vi "fpga_transmission_control_3V10.vi"() -> ()   [LabVIEW 2017]
uses:
  Control 1.ctl
  <vilib>/Platform/TimedLoop/XDataNode/timing_clust.ctl
  <vilib>/Platform/TimedLoop/XDataNode/nitl_modes.ctl
  <vilib>/Platform/TimedLoop/XDataNode/wakeup.ctl
  <vilib>/Instr/_visa.llb/VISA Configure Serial Port (Serial Instr).vi
  <vilib>/platform/TimedLoop/XDataNode/XDataNode.xnode
  <vilib>/Platform/TimedLoop/XDataNode/XDNodeRunTimeDep.lvlib
panel:
  out "Timer":dbl
  out "Output":bool
  out "outcome":u32
  out "currentType":string
  out "Time":dbl(slide) scale=0.0..100.0
  out "Progress":dbl(slide) scale=0.0..100.0
  in  "error in (no error)":errorcluster
  out "PWM":bool
  out "pattern":u32
  in  "Timeslot":bool
  out "type":string
  out "Kombi Chart":cluster{u16, i16}(graph)
  out "contingency":string
  in  "Array":T2(array[cluster]) {"duration" step=1}
  out "Timeslot":i32
  out "Sign":bool
  out "deleted portion":u8[](array[numeric])
  out "data":bool
  out "x-y":u16
  out "Error String":string
  out "error out":errorcluster
  out "Timing":u32
  out "Int_pixel":i16
  out "Pixel":u16(graph)
  out "AD_Value":i16
  in  "millisecond timer value 2":u32
  out "AD_Chart":i16(graph)
  in  "Path":path
  out "Read":bool
  in  "Stop Program":bool
  in  "Start":bool
  in  "VISA resource name":refnum<visa-resource-name>
  # "UR Elektronik Biologie\nTerminal V 3.8"
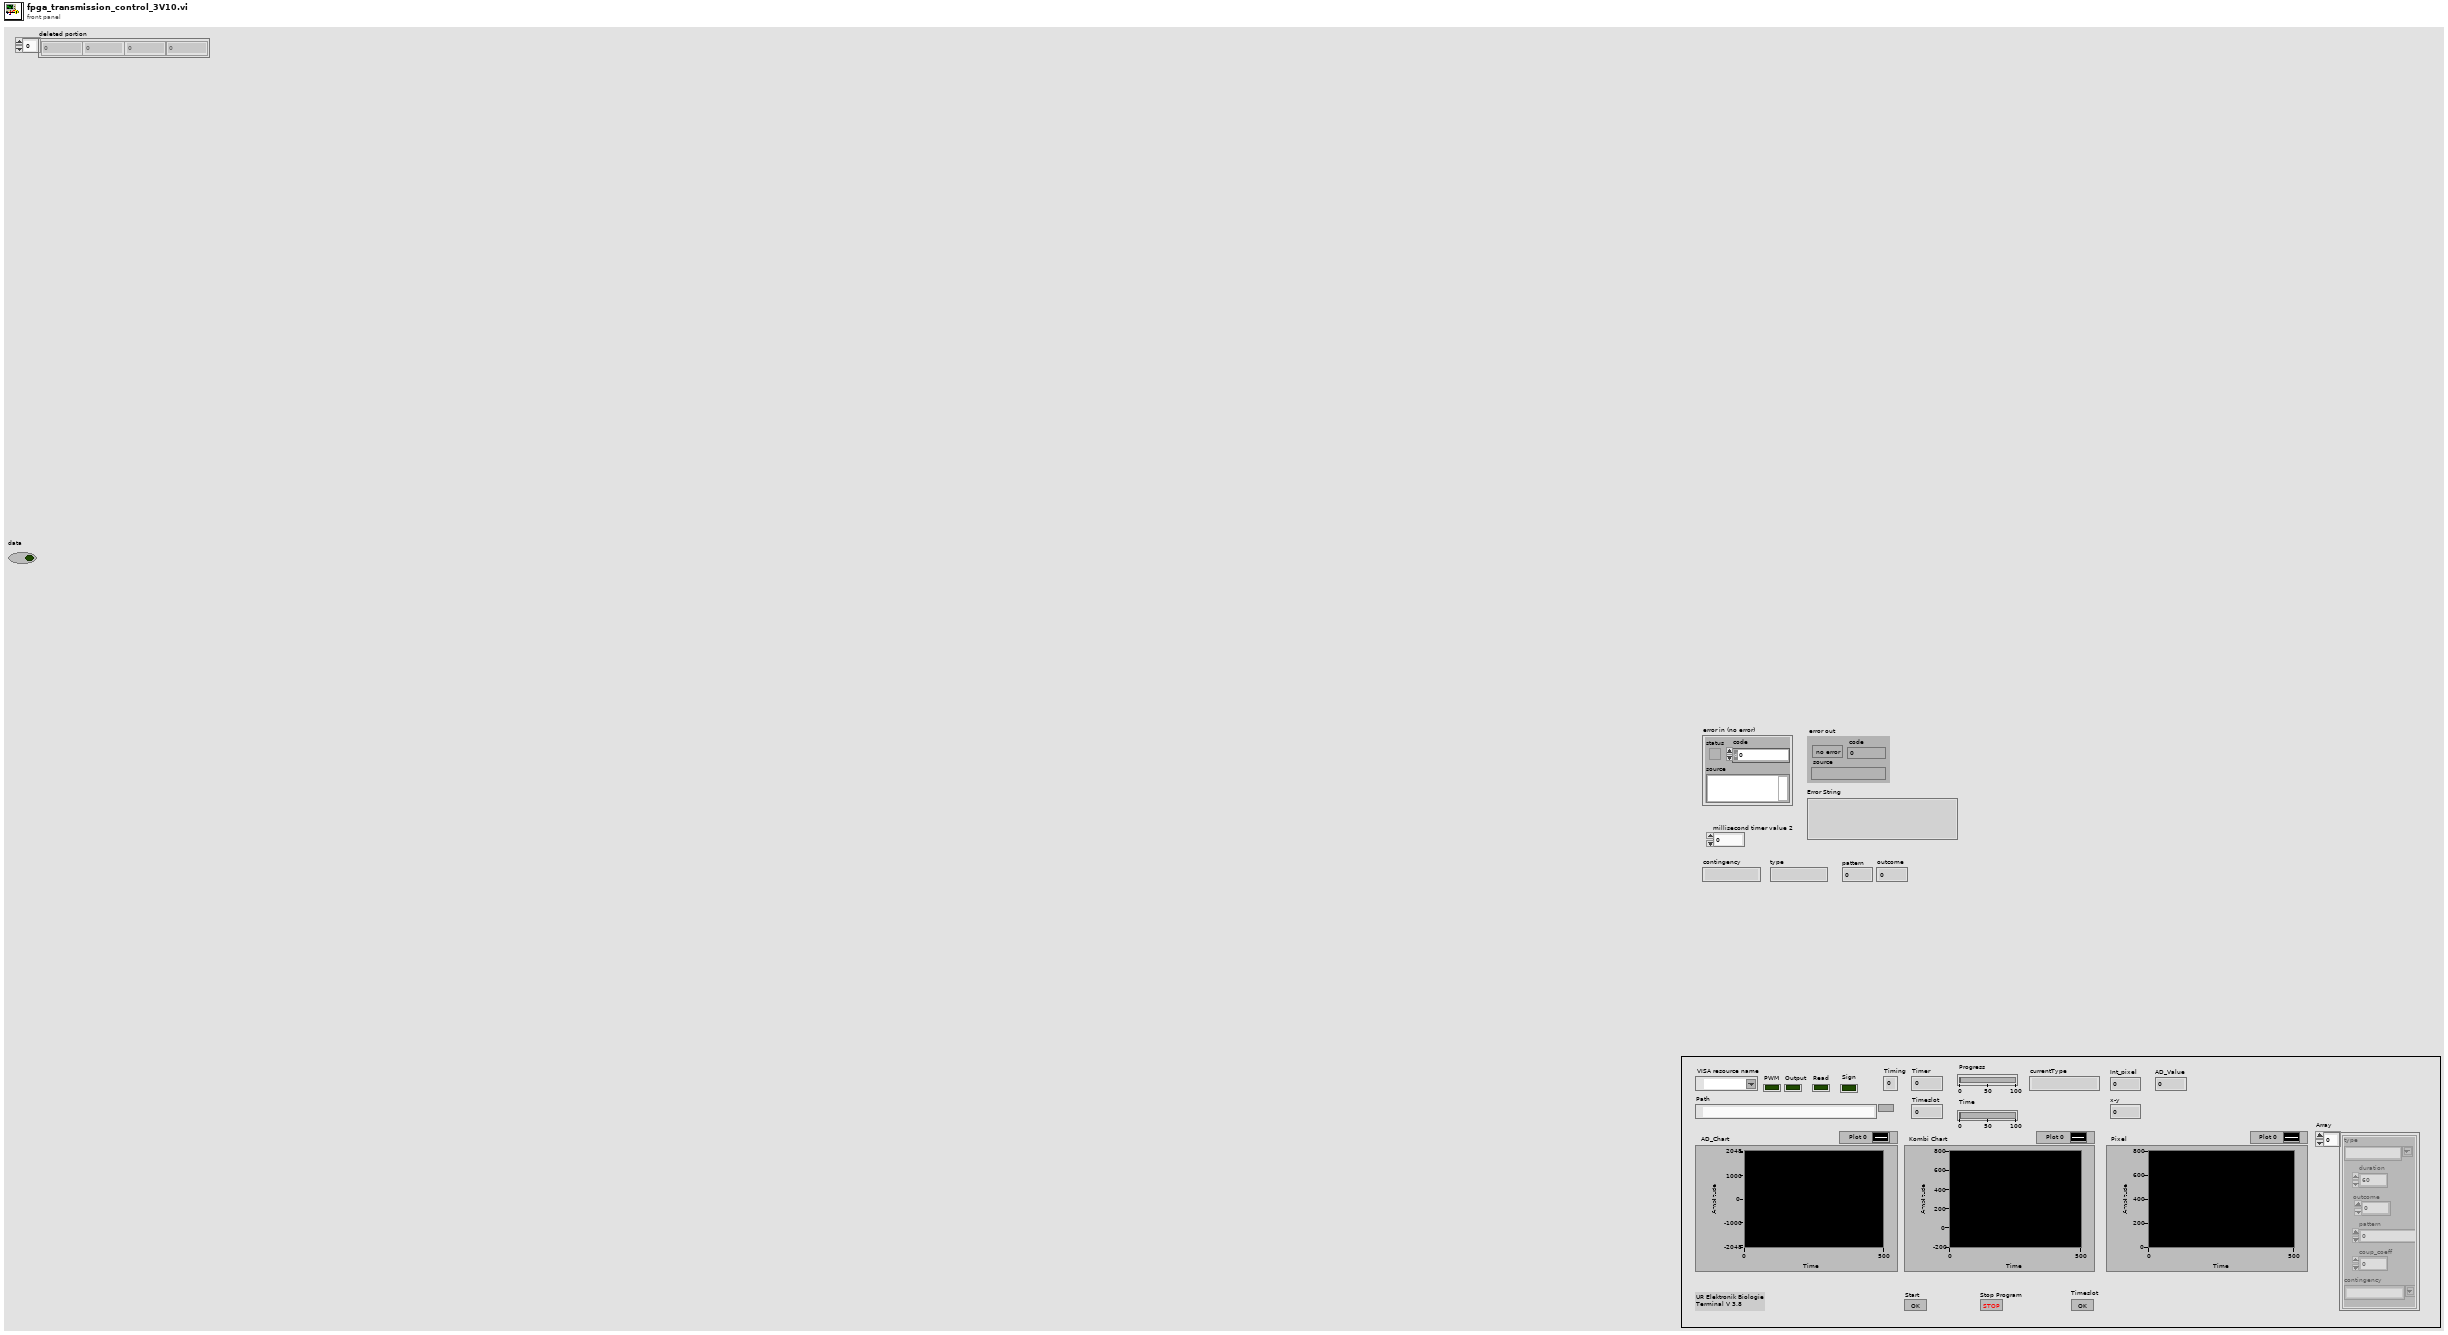
[diagram p1: front panel]
types:
  T1 = typedef "Control 1.ctl" = u32
  T2 = cluster{"type":string, "duration":T1, "outcome":u32, "pattern":u32, "coup_coeff":u32, "contingency":string}[]
  T3 = typedef "XDNodeRunTimeDep.lvlib/timing_clust.ctl" = cluster{"Expected End [f-1]":u64, "Actual End [f-1]":u64, "Finished Late? [f-1]":bool, "Expected End [i-1]":u64, "Actual End [i-1]":u64, "Finished Late? [i-1]":bool, "Expected Start [i]":u64, "Actual Start [i]":u64, "Expected Start [f]":u64, "Actual Start [f]":u64, "Source Name":string, "Structure Name":string, "Period":i64, "Deadline":i64, "Offset":i64, "Start":i64, "Priority":i32, "Timeout":i32, "Mode":T4, "Wakeup Reason":T5, "Error":errorcluster, "Source Type":string, "Secondary Source Type":string, "Global End Time":u64, "Global Start Time":u64, "Frame Duration":u64, "Iteration Duration":u64, "Assigned CPU":i32, "I/O Scan Engine Mode":u32}
  T4 = typedef "XDNodeRunTimeDep.lvlib/nitl_modes.ctl" = enum32{"No Change", "Process missed periods, maintain original phase", "Discard missed periods, maintain original phase", "Process missed periods, ignore original phase", "Discard missed periods, ignore original phase"}
  T5 = typedef "XDNodeRunTimeDep.lvlib/wakeup.ctl" = enum32{"Normal", "Aborted", "Asynchronous wakeup", "Timing source error", "Timed loop error", "Timeout"}
  T6 = cluster{"String":string, i32, i32, u32, u32, "String":string}[]
  T7 = enum16{"Idel", "State1", "State2", "State3", "State4"}
  T8 = enum16{"open", "replace", "create", "open or create", "replace or create", "replace or create with confirmation"}
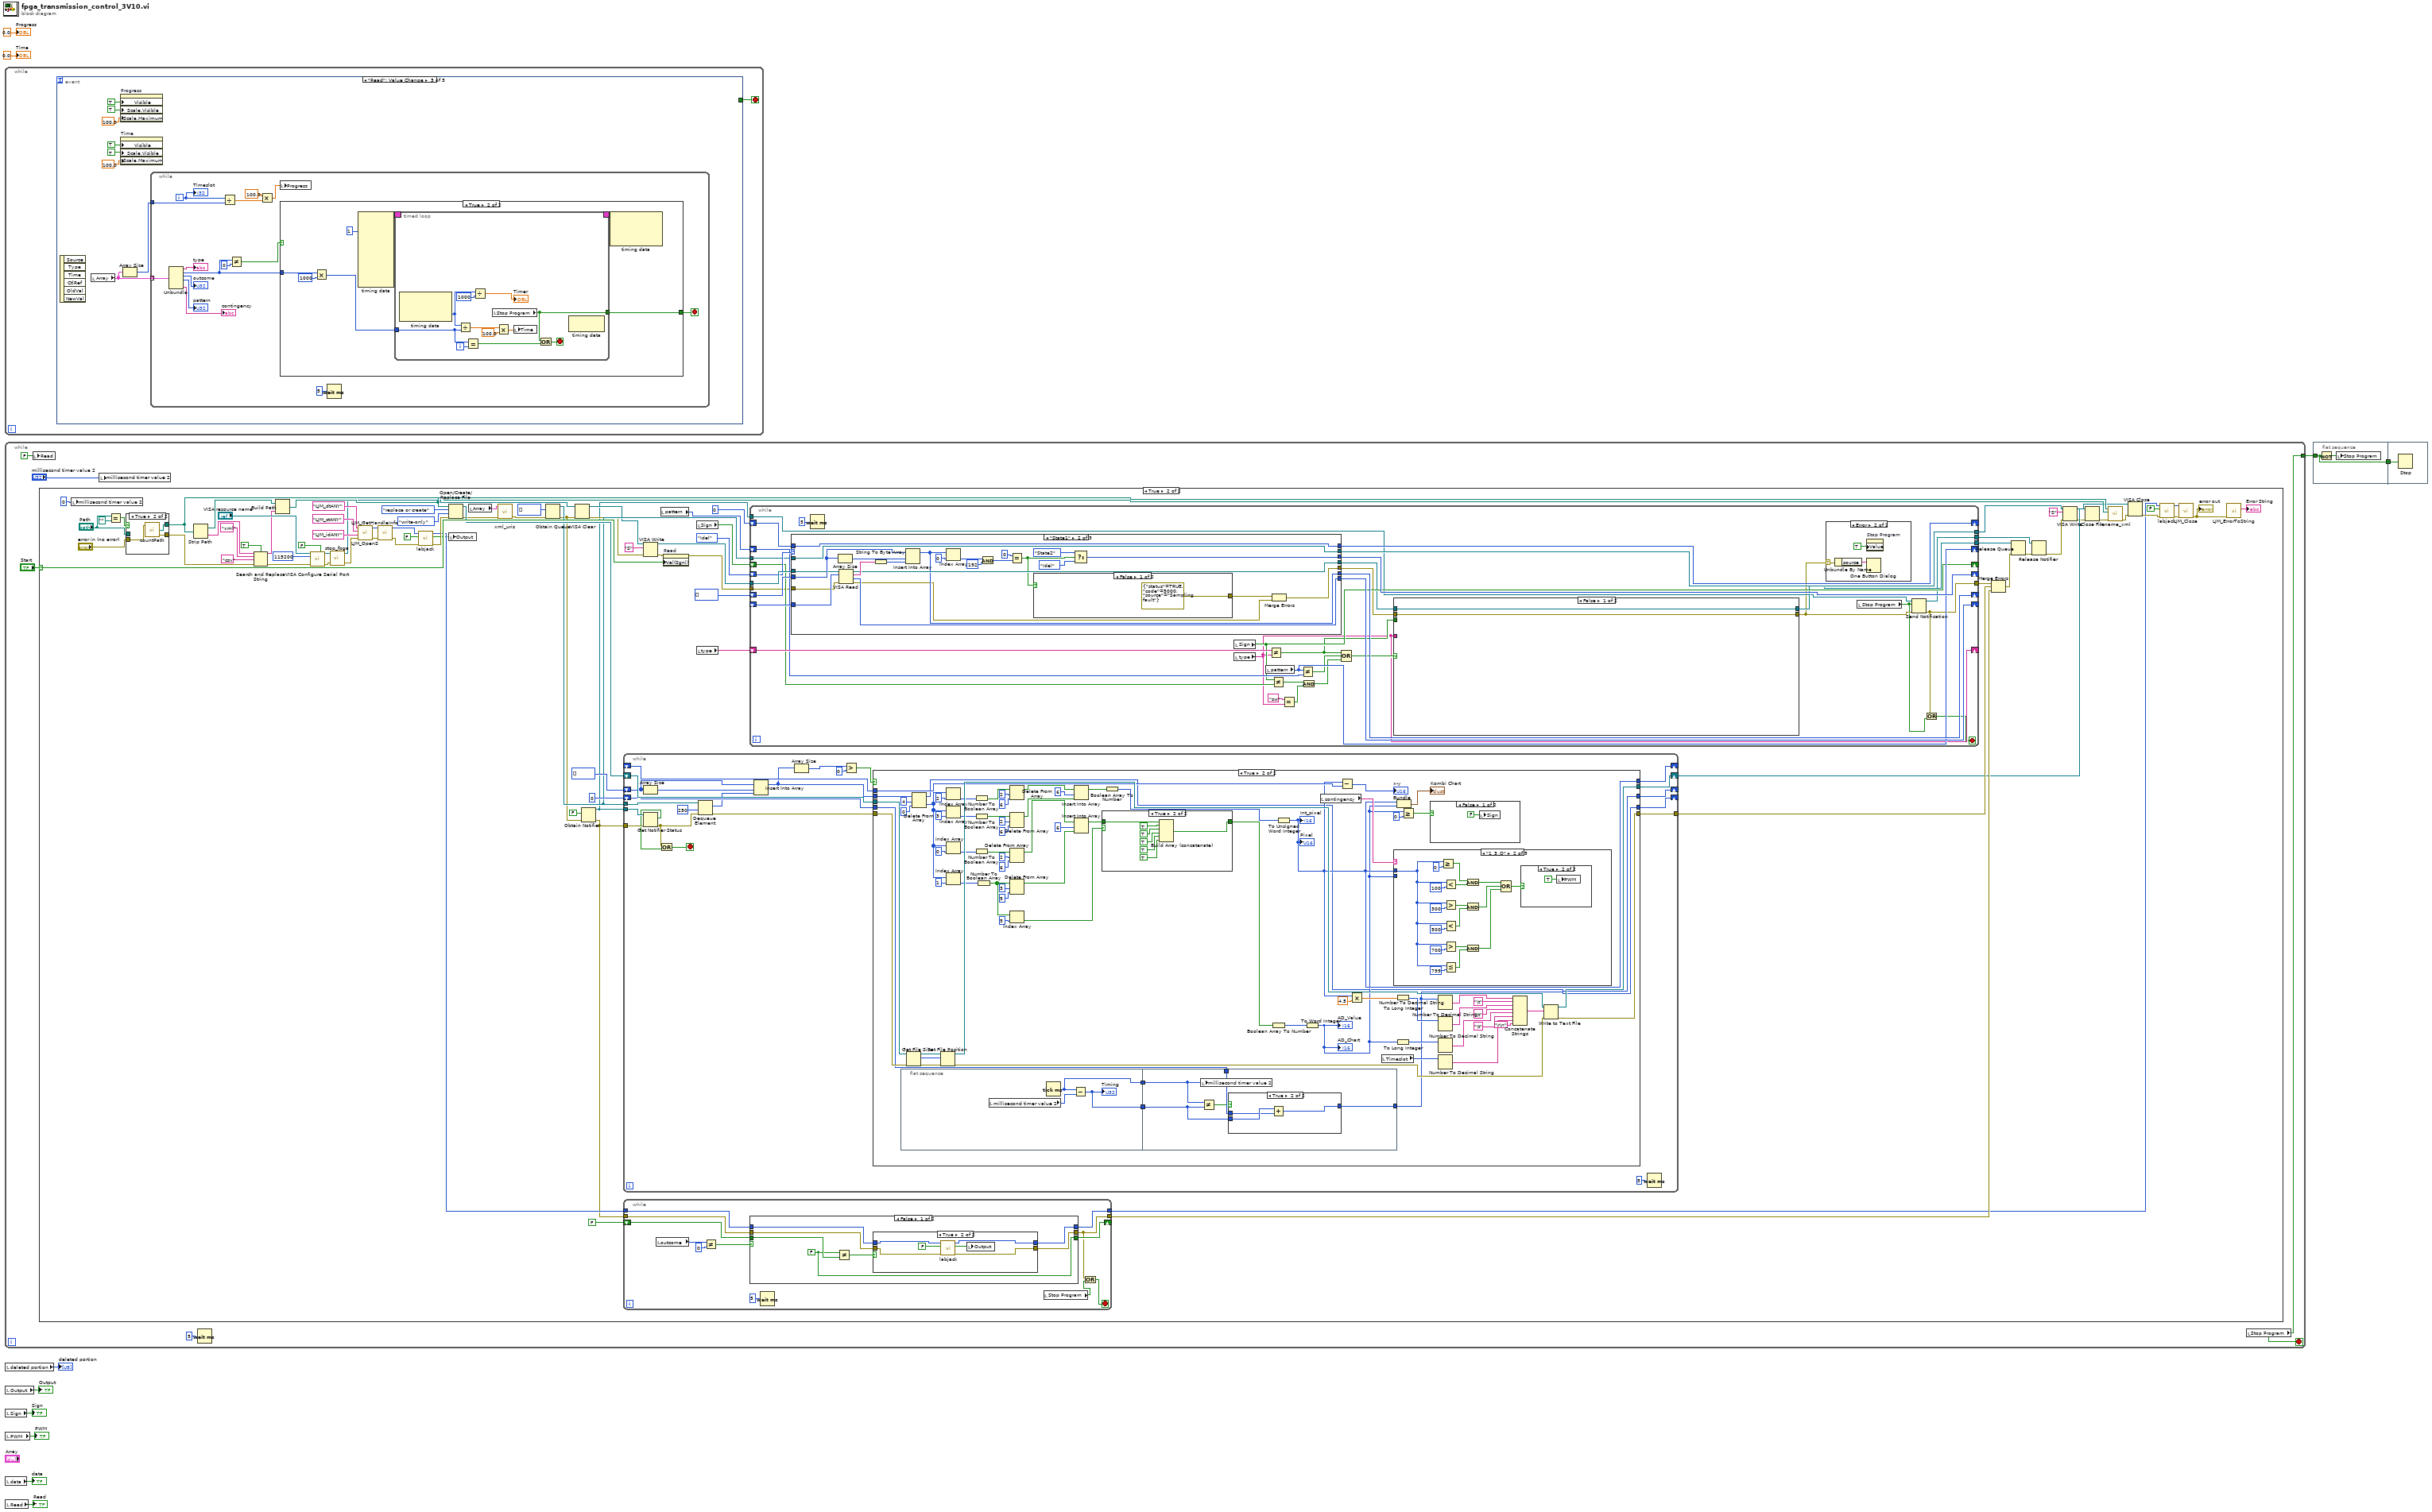
[diagram p0: block diagram]
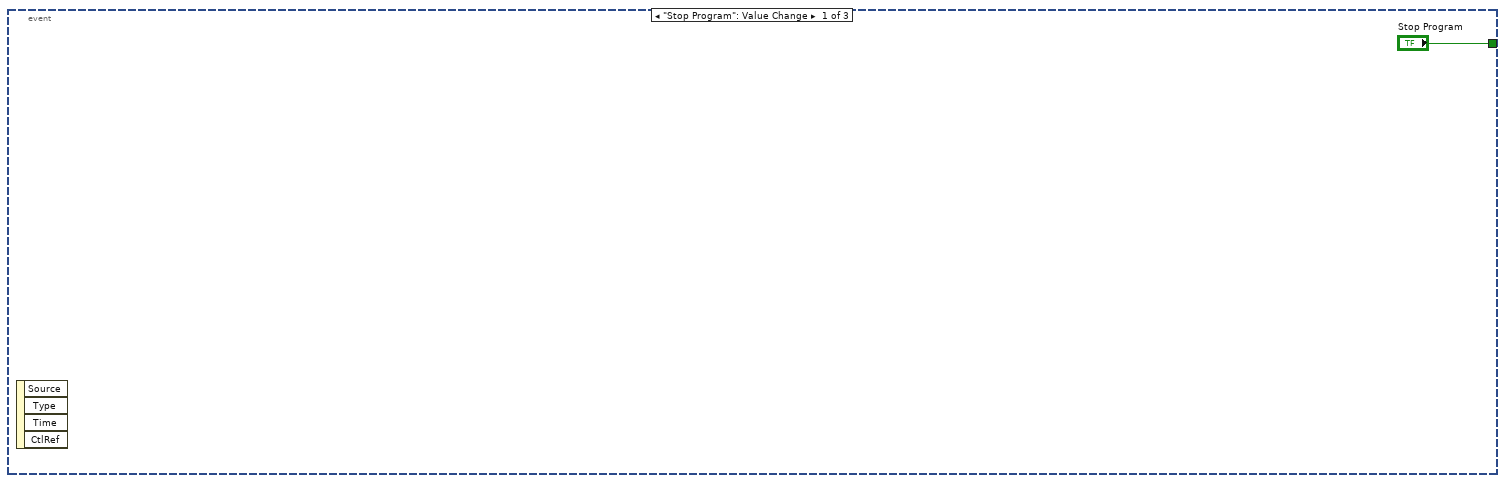
[diagram p2: hidden frame]
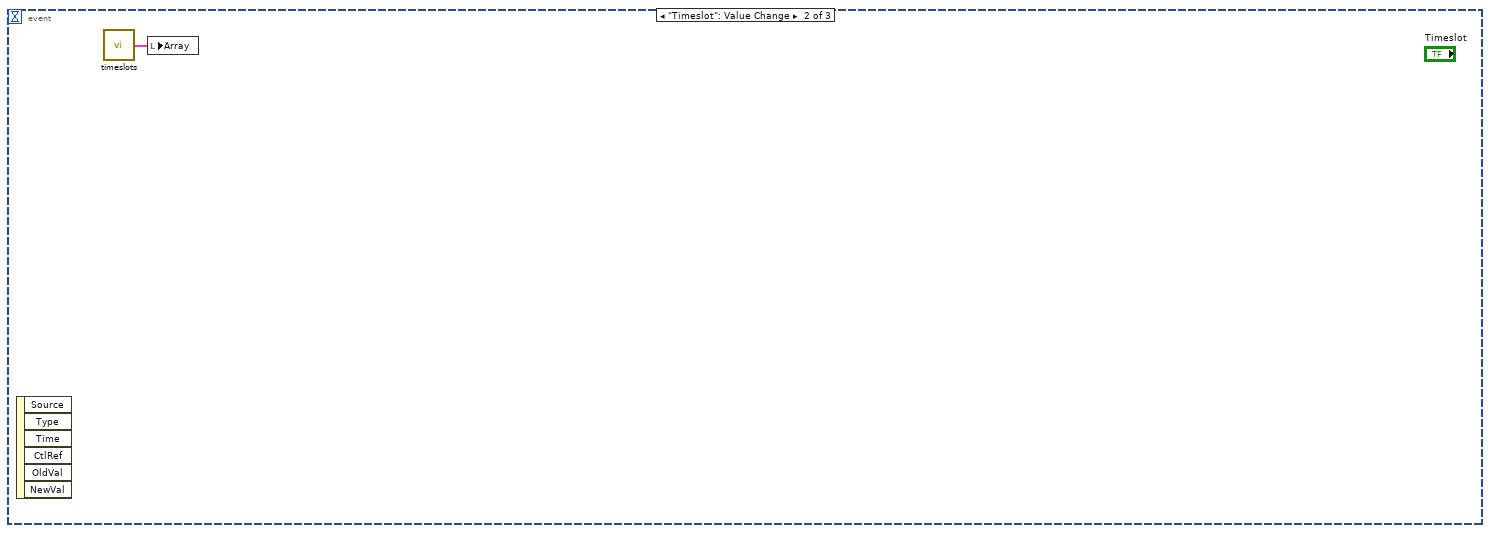
[diagram p3: hidden frame]
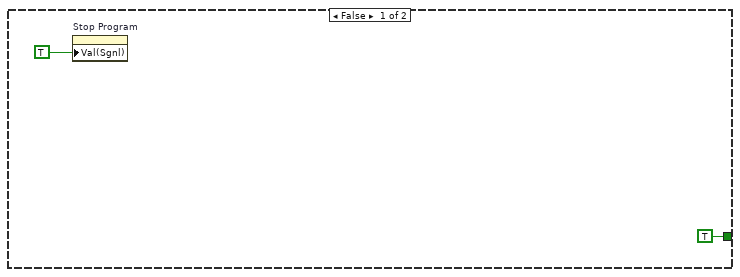
[diagram p4: hidden frame]
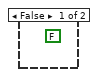
[diagram p5: hidden frame]
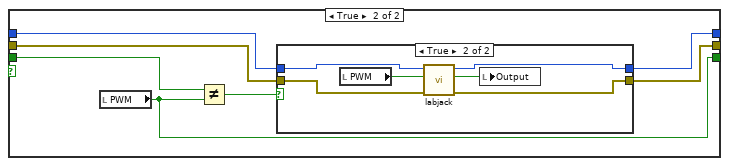
[diagram p8: hidden frame]
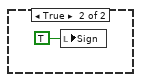
[diagram p11: hidden frame]
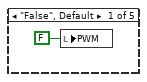
[diagram p12: hidden frame]
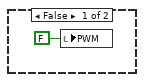
[diagram p13: hidden frame]
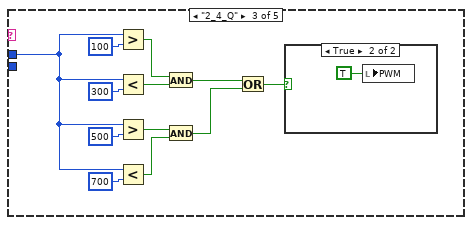
[diagram p14: hidden frame]
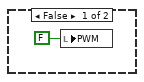
[diagram p15: hidden frame]
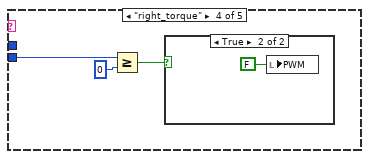
[diagram p16: hidden frame]
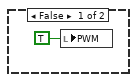
[diagram p17: hidden frame]
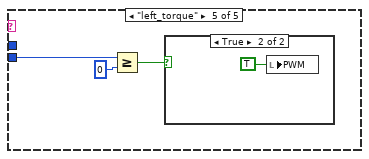
[diagram p18: hidden frame]
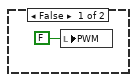
[diagram p19: hidden frame]
diagram:
  n1 = while {
    stop <- w11 stop-if-true
    n2 = event shown="[2] \"Read\": Value Change" {
      selector: _ -> [_ _ _]
      dyn-events: _ -> [_ _ _]
      timeout: _ -> [_ _ _]
      tunnel: ["Stop Program" _ _] -> w11
      event "Stop Program": Value Change {
        n3 = event-data() -> ()  [unwired: 1 in, 4 out]
      }
      event "Timeslot": Value Change {
        n4 = event-data() -> ()  [unwired: 1 in, 6 out]
        n5 = call "timeslots.vi"() -> ("array of clusters"=w13:T6)  [unwired: 1 in, 1 out]
        n6 = local write "Array"(w13) -> ()
      }
      event "Read": Value Change {
        n7 = event-data() -> ()  [unwired: 1 in, 6 out]
        n8 = local read "Array"() -> (w21:T2)
        n9 = property on="Progress" class="Slide (strict)"("Visible"=TRUE, "Scale.Visible"=TRUE ("Visible"), "Scale.Maximum"=100.0 ("Scale.Range:Maximum")) -> ()  [unwired: 2 in, 2 out]
        n10 = property on="Time" class="Slide (strict)"("Visible"=TRUE, "Scale.Visible"=TRUE ("Visible"), "Scale.Maximum"=100.0 ("Scale.Range:Maximum")) -> ()  [unwired: 2 in, 2 out]
        n11 = Array Size(array=w21) -> (size(s)=w20:i32)
        n12 = while {
          tunnel: w21 -> [w36] mode=indexing
          tunnel: w20 -> [w29]
          i -> [w28]
          stop <- w22 stop-if-true
          n13 = Unbundle(w36) -> ("type"=→"type":string, "duration"=w23:T1, "outcome"=→"outcome":u32, "pattern"=→"pattern":u32, "contingency"=→"contingency":string)  [unwired: 1 out]
          n14 = Divide(x=w28, y=w29) -> (x/y=w27:dbl)
          n15 = Not Equal?(x=w23, y=u32 0) -> (x != y?=w34:bool)
          n16 = Multiply(x=100.0 ("y"), y=w27) -> (x*y=w25:dbl)
          n17 = local write "Progress"(w25) -> ()
          n18 = case shown="True" w34 {
            tunnel: w23 -> [_ w42]
            tunnel: [TRUE w39] -> w22
            frame False {
              n19 = property on="Stop Program" class="Bool (strict)"("Val(Sgnl)"=TRUE) -> ()  [unwired: 2 in, 2 out]
            }
            frame True {
              n20 = Multiply(x=w42, y=T1 1000) -> (x*y=w40:T1)
              n21 = node-c288(i64 1 ("Period")) -> (w45:T3)  [unwired: 8 in]
              n22 = timed-loop {
                timing: w45 -> [_]
                timing-out: [_] -> w44
                tunnel: w40 -> [w52]
                tunnel: [w53] -> w39
                i -> [w56]
                stop <- w55 stop-if-true
                n23 = node-c288() -> (w48:i64)  [unwired: 1 in, 2 out]
                n24 = Divide(x=w48, y=w52) -> (x/y=w50:dbl)
                n25 = Equal?(x=w52, y=w56) -> (x = y?=w54:bool)
                n26 = Divide(x=w48, y=i64 1000) -> (x/y=→"Timer":dbl)
                n27 = local read "Stop Program"() -> (w53:bool)
                n28 = Multiply(x=w50, y=100.0) -> (x*y=w51:dbl)
                n29 = local write "Time"(w51) -> ()
                n30 = Or(x=w53, y=w54) -> (x .or. y?=w55:bool)
                n31 = node-c288() -> ()  [unwired: 1 in, 1 out]
              }
              n32 = node-c288(w44) -> ()  [unwired: 3 out]
            }
          }
          n33 = Wait (ms)(milliseconds to wait=u32 5) -> ()  [unwired: 1 out]
          "Timeslot" <- w28
        }
      }
    }
  }
  n34 = while {
    tunnel: [w67] -> w10
    stop <- w67 stop-if-true
    n35 = local write "Read"(FALSE) -> ()
    n36 = case shown="True" "Start" {
      selector: "Start" -> [_ w145]
      frame False {
        (unwired) FALSE
      }
      frame True {
        n37 = local write "millisecond timer value 2"(u32 0 ("millisecond timer value 2")) -> ()
        n38 = Equal?(x="Path", y=path "") -> (x = y?=w132:bool)
        n39 = case shown="True" w132 {
          tunnel: [w153 w156] -> w98
          tunnel: "Path" -> [w153 _]
          tunnel: [w152 w155] -> w107
          tunnel: "error in (no error)" -> [w152 w154]
          frame False {
          }
          frame True {
            n40 = call "countPath.vi"("error in (no error)"=w154) -> ("error out"=w155:errorcluster, "appended path"=w156:path)
          }
        }
        n41 = Strip Path(path=w98) -> (stripped path=w111:path, name=w110:string)
        n42 = Search and Replace String(case sensitive?=TRUE ("ignore case? (F)"), input string=w110, search string="xml", replace string="csv" ("replace string (\"\")"), error in=w107) -> (result string=w104:string, error out=w106:errorcluster)  [unwired: 3 in, 2 out]
        n43 = Build Path(base path=w111, name or relative path=w104) -> (appended path=w99:path)
        n44 = call-poly "VISA Configure Serial Port"("VISA resource name"="VISA resource name", "Enable Termination\nChar (T)"=FALSE ("Enable Termination\nChar (T)"), "baud rate (9600)"=u32 115200, "error in (no error)"=w106) -> ("VISA resource name out"=w91:refnum<visa-resource-name>, "error out"=w90:errorcluster)  [unwired: 10 in]
        n45 = call "stop_fpga.vi"("error in (no error)"=w90, "reference"=w91) -> ("error out"=w89:errorcluster, "VISA resource name out"=w82:refnum<visa-resource-name>)  [unwired: 2 in]
        n46 = call "LJM_OpenS.vi"("error in"=w89, "Identifier"="LJM_idANY", "ConnectionType"="LJM_ctANY", "DeviceType"="LJM_dtANY") -> ("error out"=w135:errorcluster, "Handle"=w134:i32)  [unwired: 6 in]
        n47 = call "LJM_GetHandleInfo.vi"("error in"=w135, "Handle In"=w134) -> ("error out"=w137:errorcluster, "Handle Out"=w136:i32)  [unwired: 2 in, 6 out]
        n48 = call "labjack.vi"("error out"=w137, "Boolean"=FALSE, "Handle Out"=w136) -> ("error out 2"=w140:errorcluster, "Boolean 2"=w97:bool, "Handle Out 2"=w139:i32)  [unwired: 6 in]
        n49 = Open/Create/Replace File(file path (use dialog)=w99, error in=w140, operation (0:open)=T8."replace or create", access (0:read/write)=enum16{"read/write", "read-only", "write-only"}."write-only") -> (refnum out=w114:refnum<file>, error out=w112:errorcluster)  [unwired: 2 in, 1 out]
        n50 = local write "Output"(w97) -> ()
        n51 = local read "Array"() -> (w113:T2)
        n52 = call "xml_uris.vi"("error in"=w112, "Array"=w113) -> ("error out"=w83:errorcluster)  [unwired: 2 in, 2 out]
        n53 = Obtain Queue(element data type=u8[] [], error in (no error)=w83) -> (queue out=w85:refnum<queue>, error out=w70:errorcluster)  [unwired: 3 in, 1 out]
        n54 = VISA Clear(VISA resource name=w82, error in (no error)=w70) -> (VISA resource name out=w81:refnum<visa-resource-name>, error out=w79:errorcluster)
        n55 = Obtain Notifier(notification data type=FALSE, error in (no error)=w70) -> (notifier out=w76:refnum<notifier>, error out=w69:errorcluster)  [unwired: 2 in, 1 out]
        n56 = while {
          shift-right: [w221] -> w102
          shift-left: w114 -> [w222]
          shift-right: [w219] -> _
          shift-left: _ -> [w220]
          shift-right: [w217] -> _
          shift-left: u32 0 -> [w216]
          shift-right: [w213] -> _
          shift-left: u8[] [] -> [w214]
          tunnel: w85 -> [w202]
          tunnel: w76 -> [w205]
          tunnel: w69 -> [w204]
          tunnel: [w218] -> w103
          stop <- w201 stop-if-true
          n57 = Array Size(array=w214) -> (size(s)=w212:i32)
          n58 = Get Notifier Status(notifier=w205, error in (no error)=w204) -> (current notification=w199:bool, error out=w200:errorcluster)  [unwired: 3 out]
          n59 = Or(x=w200, y=w199) -> (x .or. y?=w201:bool)
          n60 = Dequeue Element(queue=w202, timeout in ms (-1)=250, error in (no error)=w200) -> (element=w209:u8[], error out=w206:errorcluster)  [unwired: 2 out]
          n61 = Insert Into Array(array=w214, index=w212, new element=w209) -> (w208:u8[])
          n62 = Array Size(array=w208) -> (size(s)=w207:i32)
          n63 = Greater?(x=w207, y=0) -> (0:w210:bool)
          n64 = case shown="True" w210 {
            tunnel: w206 -> [w227 w251]
            tunnel: [w227 w295] -> w218
            tunnel: w222 -> [w226 w257]
            tunnel: [w226 w294] -> w221
            tunnel: [w225 w234] -> w219
            tunnel: w220 -> [w225 w252]
            tunnel: [w224 w238] -> w217
            tunnel: w216 -> [w224 w239]
            tunnel: w208 -> [w223 w232]
            tunnel: [w223 w228] -> w213
            frame False {
            }
            frame True {
              n65 = flat-sequence {
                tunnel: [w356] -> w293
                tunnel: [w355] -> w240
                tunnel: w293 -> [w359]
                tunnel: w240 -> [w360]
                tunnel: [w362] -> w238
                tunnel: w239 -> [w361]
                frame #0 {
                  n66 = local read "millisecond timer value 2"() -> (w357:u32)
                  n67 = Tick Count (ms)() -> (millisecond timer value=w356:u32)
                  n68 = Subtract(x=w356, y=w357) -> (x-y=w355:u32)
                  "Timing" <- w355
                }
                frame #1 {
                  n69 = local write "millisecond timer value 2"(w359) -> ()
                  n70 = Not Equal?(x=w359, y=w360) -> (x != y?=w358:bool)
                  n71 = case shown="True" w358 {
                    tunnel: w360 -> [_ w366]
                    tunnel: [u32 0 w365] -> w362
                    tunnel: w361 -> [_ w364]
                    frame False {
                    }
                    frame True {
                      n72 = Add(x=w366, y=w364) -> (x+y=w365:u32)
                    }
                  }
                }
              }
              n73 = Get File Size(file=w257, error in=w251) -> (refnum out=w300:refnum<file>, size (in bytes)=w299:i64, 0:w298:errorcluster)
              n74 = Delete From Array(array=w232, length=4, index=0) -> (deleted portion=w229:u8[], array with subset deleted=w228:u8[])
              n75 = Set File Position(offset (in bytes) (0)=w299, refnum=w300, error in=w298) -> (refnum out=w296:refnum<file>, error out=w297:errorcluster)  [unwired: 1 in]
              n76 = Index Array(array=w229, index=2) -> (element=w254:u8)
              n77 = Index Array(array=w229, index=3) -> (element=w253:u8)
              n78 = Index Array(array=w229, index=0) -> (element=w256:u8)
              n79 = Index Array(array=w229, index=1) -> (element=w255:u8)
              n80 = Number To Boolean Array(number=w254) -> (Boolean array=w275:bool[])
              n81 = Number To Boolean Array(number=w253) -> (Boolean array=w278:bool[])
              n82 = Number To Boolean Array(number=w256) -> (Boolean array=w265:bool[])
              n83 = Number To Boolean Array(number=w255) -> (Boolean array=w284:bool[])
              n84 = Delete From Array(array=w275, length=2, index=6 ("length")) -> (array with subset deleted=w288:bool[])  [unwired: 1 out]
              n85 = Delete From Array(array=w278, length=2, index=6) -> (array with subset deleted=w289:bool[])  [unwired: 1 out]
              n86 = Delete From Array(array=w265, length=2, index=6 ("length")) -> (array with subset deleted=w268:bool[])  [unwired: 1 out]
              n87 = Delete From Array(array=w284, length=3, index=5) -> (array with subset deleted=w273:bool[])  [unwired: 1 out]
              n88 = Index Array(array=w284, index=5) -> (element=w286:bool)
              n89 = Insert Into Array(array=w288, index=6, new element=w289) -> (w282:bool[])
              n90 = Insert Into Array(array=w268, index=6, new element=w273) -> (w270:bool[])
              n91 = case shown="True" w286 {
                tunnel: w270 -> [w347 w354]
                tunnel: [w347 w349] -> w287
                frame False {
                }
                frame True {
                  n92 = Build Array (concatenate)(w354, TRUE ("new element/subarray"), TRUE ("new element/subarray"), TRUE ("new element/subarray"), TRUE ("new element/subarray"), TRUE ("element")) -> (w349:bool[])
                }
              }
              n93 = Boolean Array To Number(Boolean array=w282) -> (number=w283:u32)
              n94 = Boolean Array To Number(Boolean array=w287) -> (number=w274:u32)
              n95 = To Unsigned Word Integer(number=w283) -> (unsigned 16bit integer=w234:u16)
              "Pixel" <- w234
              "Int_pixel" <- w234
              n96 = To Word Integer(number=w274) -> (16bit integer=w233:i16)
              "AD_Chart" <- w233
              "AD_Value" <- w233
              n97 = local read "contingency"() -> (w241:string)
              n98 = Subtract(x=w234, y=w252) -> (x-y=→"x-y":u16)
              n99 = Multiply(x=w234, y=4.5) -> (x*y=w243:dbl)
              n100 = local read "Timeslot"() -> (w247:i32)
              n101 = case shown="\"1_3_Q\"" w241 {
                tunnel: w234 -> [_ w305 w331 _ _]
                tunnel: w233 -> [_ _ _ w337 w342]
                frame "False", Default {
                  n102 = local write "PWM"(FALSE ("pwm")) -> ()
                }
                frame "1_3_Q" {
                  n103 = Greater Or Equal?(x=w305, y=u16 0 ("x")) -> (x >= y?=w304:bool)
                  n104 = Less?(x=w305, y=u16 100) -> (x < y?=w315:bool)
                  n105 = Greater?(x=w305, y=u16 300 ("a")) -> (0:w317:bool)
                  n106 = Less?(x=w305, y=u16 500 ("b")) -> (x < y?=w316:bool)
                  n107 = Greater?(x=w305, y=u16 700) -> (0:w314:bool)
                  n108 = Less Or Equal?(x=w305, y=u16 799) -> (x <= y?=w312:bool)
                  n109 = And(x=w304, y=w315) -> (x .and. y?=w310:bool)
                  n110 = And(x=w317, y=w316) -> (x .and. y?=w309:bool)
                  n111 = And(x=w314, y=w312) -> (x .and. y?=w308:bool)
                  n112 = Compound Arithmetic op=OR(w310, w309, w308) -> (w307:bool)
                  n113 = case shown="True" w307 {
                    frame False {
                      n114 = local write "PWM"(FALSE ("pwm")) -> ()
                    }
                    frame True {
                      n115 = local write "PWM"(TRUE ("pwm")) -> ()
                    }
                  }
                }
                frame "2_4_Q" {
                  n116 = Greater?(x=w331, y=u16 100 ("x")) -> (0:w326:bool)
                  n117 = Less?(x=w331, y=u16 300) -> (x < y?=w327:bool)
                  n118 = Greater?(x=w331, y=u16 500 ("a")) -> (0:w330:bool)
                  n119 = Less?(x=w331, y=u16 700 ("b")) -> (x < y?=w328:bool)
                  n120 = And(x=w326, y=w327) -> (x .and. y?=w325:bool)
                  n121 = And(x=w330, y=w328) -> (x .and. y?=w329:bool)
                  n122 = Or(x=w325, y=w329) -> (x .or. y?=w324:bool)
                  n123 = case shown="True" w324 {
                    frame False {
                      n124 = local write "PWM"(FALSE ("pwm")) -> ()
                    }
                    frame True {
                      n125 = local write "PWM"(TRUE ("pwm")) -> ()
                    }
                  }
                }
                frame "right_torque" {
                  n126 = Greater Or Equal?(x=w337, y=i16 0) -> (x >= y?=w338:bool)
                  n127 = case shown="True" w338 {
                    frame False {
                      n128 = local write "PWM"(TRUE ("pwm")) -> ()
                    }
                    frame True {
                      n129 = local write "PWM"(FALSE ("pwm")) -> ()
                    }
                  }
                }
                frame "left_torque" {
                  n130 = Greater Or Equal?(x=w342, y=i16 0) -> (x >= y?=w343:bool)
                  n131 = case shown="True" w343 {
                    frame False {
                      n132 = local write "PWM"(FALSE ("pwm")) -> ()
                    }
                    frame True {
                      n133 = local write "PWM"(TRUE ("pwm")) -> ()
                    }
                  }
                }
              }
              n134 = To Long Integer(number=w243) -> (32bit integer=w242:i32)
              n135 = To Long Integer(number=w233) -> (32bit integer=w245:i32)
              n136 = Bundle(w234, w233) -> (→"Kombi Chart":cluster{u16, i16})  [unwired: 1 in]
              n137 = Greater Or Equal?(x=w233, y=i16 0) -> (x >= y?=w235:bool)
              n138 = case shown="False" w235 {
                frame False {
                  n139 = local write "Sign"(FALSE) -> ()
                }
                frame True {
                  n140 = local write "Sign"(TRUE) -> ()
                }
              }
              n141 = Number To Decimal String(number=w238) -> (decimal integer string=w250:string)  [unwired: 1 in]
              n142 = Number To Decimal String(number=w242) -> (decimal integer string=w290:string)  [unwired: 1 in]
              n143 = Number To Decimal String(number=w245) -> (decimal integer string=w248:string)  [unwired: 1 in]
              n144 = Number To Decimal String(number=w247) -> (decimal integer string=w246:string)  [unwired: 1 in]
              n145 = Concatenate Strings(w250, "\t" ("string"), w290, "\t" ("string"), w248, "\t" ("string"), w246, "\r\n") -> (w258:string)
              n146 = Write to Text File(file (use dialog)=w296, text=w258, error in=w297) -> (refnum out=w294:refnum<file>, error out=w295:errorcluster)  [unwired: 1 in, 1 out]
            }
          }
          n147 = Wait (ms)(milliseconds to wait=u32 5) -> ()  [unwired: 1 out]
        }
        n148 = while {
          tunnel: w139 -> [w167]
          tunnel: w69 -> [w166]
          shift-right: [w164] -> _
          shift-left: FALSE ("pwm") -> [w168]
          tunnel: [w165] -> w121
          tunnel: [w157] -> w146
          stop <- w158 stop-if-true
          n149 = local read "outcome"() -> (w163:u32)
          n150 = Not Equal?(x=w163, y=u32 0) -> (x != y?=w161:bool)
          n151 = case shown="False" w161 {
            tunnel: w168 -> [w171 w190]
            tunnel: w167 -> [w175 w185]
            tunnel: w166 -> [w173 w186]
            tunnel: [w174 w189] -> w165
            tunnel: [w172 w188] -> w157
            tunnel: [w170 w187] -> w164
            frame False {
              w170 = FALSE ("Boolean")
              n152 = Not Equal?(x=w170, y=w171) -> (x != y?=w169:bool)
              n153 = case shown="True" w169 {
                tunnel: w175 -> [w177 w183]
                tunnel: [w177 w182] -> w174
                tunnel: w173 -> [w176 w181]
                tunnel: [w176 w180] -> w172
                frame False {
                }
                frame True {
                  n154 = call "labjack.vi"("error out"=w181, "Boolean"=FALSE, "Handle Out"=w183) -> ("error out 2"=w180:errorcluster, "Boolean 2"=w178:bool, "Handle Out 2"=w182:i32)  [unwired: 6 in]
                  n155 = local write "Output"(w178) -> ()
                }
              }
            }
            frame True {
              n156 = local read "PWM"() -> (w187:bool)
              n157 = Not Equal?(x=w190, y=w187) -> (x != y?=w184:bool)
              n158 = case shown="True" w184 {
                tunnel: w185 -> [w192 w198]
                tunnel: w186 -> [w191 w197]
                tunnel: [w192 w196] -> w189
                tunnel: [w191 w195] -> w188
                frame False {
                }
                frame True {
                  n159 = local read "PWM"() -> (w194:bool)
                  n160 = call "labjack.vi"("error out"=w197, "Boolean"=w194, "Handle Out"=w198) -> ("error out 2"=w195:errorcluster, "Boolean 2"=w193:bool, "Handle Out 2"=w196:i32)  [unwired: 6 in]
                  n161 = local write "Output"(w193) -> ()
                }
              }
            }
          }
          n162 = Wait (ms)(milliseconds to wait=u32 5) -> ()  [unwired: 1 out]
          n163 = local read "Stop Program"() -> (w159:bool)
          n164 = Or(x=w157, y=w159) -> (x .or. y?=w158:bool)
        }
        n165 = VISA Write(VISA resource name=w81, write buffer="S", error in (no error)=w79) -> (VISA resource name out=w80:refnum<visa-resource-name>, error out=w88:errorcluster)  [unwired: 1 out]
        n166 = local read "pattern"() -> (w117:u32)
        n167 = property on="Read" class="Bool (strict)"(error in=w88, "Val(Sgnl)"=w145) -> (error out=w78:errorcluster)  [unwired: 1 in, 1 out]
        n168 = local read "Sign"() -> (w116:bool)
        n169 = local read "type"() -> (w141:string)
        n170 = while {
          tunnel: w80 -> [w401]
          shift-right: [w395] -> _
          shift-left: u8[] [] -> [w400]
          tunnel: [w377] -> w94
          shift-right: [w399] -> _
          shift-left: T7."Idel" -> [w398]
          shift-right: [w397] -> _
          shift-left: _ -> [w396]
          shift-right: [w394] -> _
          shift-left: u8 0 -> [w393]
          shift-right: [w384] -> _
          shift-left: w141 -> [w392]
          shift-right: [w391] -> _
          shift-left: w117 -> [w390]
          shift-right: [w389] -> _
          shift-left: w116 -> [w388]
          tunnel: w85 -> [w376]
          tunnel: [w375] -> w84
          tunnel: w76 -> [w372]
          tunnel: w78 -> [w373]
          tunnel: [w369] -> w73
          tunnel: [w370] -> w74
          stop <- w367 stop-if-true
          n171 = case shown="\"State1\"" w398 {
            tunnel: w401 -> [w519 w544 w564]
            tunnel: w373 -> [w520 w545 w558]
            tunnel: w400 -> [w523 w547 w571]
            tunnel: [w527 w549 w564] -> w378
            tunnel: [w526 w533 w557] -> w379
            tunnel: [w528 w546 w567] -> w399
            tunnel: [w525 w550 w565] -> w397
            tunnel: w396 -> [_ w551 w565]
            tunnel: [w523 w543 w570] -> w395
            tunnel: [w522 w542 u8 0] -> w394
            tunnel: w393 -> [w522 w542 _]
            tunnel: w376 -> [w517 w536 w560]
            tunnel: [w517 w536 w559] -> w375
            frame "Idel", Default {
              n172 = local write "data"(FALSE ("data")) -> ()
              n173 = property class="Serial Instr"(reference=w519, error in=w520) -> (reference out=w527:refnum<visa-resource-name>, error out=w526:errorcluster, "Serial Settings:Number of Bytes at Serial Port"=w525:u32)
              n174 = Greater Or Equal?(x=w525, y=u8 4) -> (x >= y?=w518:bool)
              n175 = Select(t=T7."State1", s=w518, f=T7."Idel") -> (s? t:f=w528:T7)
            }
            frame "State1" {
              n176 = Array Size(array=w547) -> (size(s)=w535:i32)
              n177 = VISA Read(VISA resource name=w544, byte count=w551, error in (no error)=w545) -> (VISA resource name out=w549:refnum<visa-resource-name>, read buffer=w552:string, return count=w550:u32, error out=w531:errorcluster)
              n178 = String To Byte Array(string=w552) -> (unsigned byte array=w548:u8[])
              n179 = Insert Into Array(array=w547, index=w535, new element=w548) -> (w543:u8[])
              n180 = Index Array(array=w543, index=0) -> (element=w540:u8)
              n181 = And(x=w540, y=u8 192) -> (x .and. y?=w539:u8)
              n182 = Equal?(x=u8 0, y=w539) -> (x = y?=w532:bool)
              n183 = case shown="False" w532 {
                tunnel: [errorcluster {"status"=TRUE, "code"=5000, "source"="Sampling fault"} ("error constant") errorcluster {"status"=FALSE, "code"=0, "source"=""} ("error constant")] -> w534
                frame False {
                }
                frame True {
                }
              }
              n184 = Select(t=T7."State2", s=w532, f=T7."Idel") -> (s? t:f=w546:T7)
              n185 = Merge Errors(w534, w531) -> (w533:errorcluster)
            }
            frame "State2" {
              n186 = Delete From Array(array=w571, length=4, index=0) -> (deleted portion=w561:u8[], array with subset deleted=w570:u8[])
              n187 = Array Size(array=w570) -> (size(s)=w569:i32)
              n188 = Enqueue Element(queue=w560, element=w561, error in (no error)=w558) -> (queue out=w559:refnum<queue>, error out=w557:errorcluster)  [unwired: 1 in, 1 out]
              n189 = Greater Or Equal?(x=w569, y=4) -> (x >= y?=w562:bool)
              n190 = Select(t=T7."State2", s=w562, f=T7."Idel") -> (s? t:f=w567:T7)
            }
          }
          n191 = Wait (ms)(milliseconds to wait=u32 5) -> ()  [unwired: 1 out]
          n192 = local read "Sign"() -> (w389:bool)
          n193 = local read "type"() -> (w384:string)
          n194 = local read "pattern"() -> (w391:u32)
          n195 = Not Equal?(x=w392, y=w384) -> (x != y?=w385:bool)
          n196 = Not Equal?(x=w389, y=w388) -> (x != y?=w381:bool)
          n197 = Equal?(x="sw", y=w384) -> (x = y?=w382:bool)
          n198 = Not Equal?(x=w391, y=w390) -> (x != y?=w387:bool)
          n199 = And(x=w381, y=w382) -> (x .and. y?=w380:bool)
          n200 = Compound Arithmetic op=OR(w385, w387, w380) -> (w386:bool)
          n201 = case shown="False" w386 {
            tunnel: w378 -> [w406 w410]
            tunnel: [w406 w413] -> w377
            tunnel: w379 -> [w405 w409]
            tunnel: [w405 w414] -> w371
            tunnel: w384 -> [_ w407]
            tunnel: w385 -> [_ w408]
            frame False {
            }
            frame True {
              n202 = case shown="True" w408 {
                tunnel: [w416 w422] -> w412
                tunnel: [w417 w421] -> w411
                tunnel: w410 -> [w417 w419]
                tunnel: w409 -> [w416 w418]
                frame False {
                }
                frame True {
                  n203 = VISA Write(VISA resource name=w419, write buffer="1W", error in (no error)=w418) -> (VISA resource name out=w421:refnum<visa-resource-name>, error out=w422:errorcluster)  [unwired: 1 out]
                }
              }
              n204 = case shown="\"fs\"" w407 {
                tunnel: w411 -> [w424 w431 w436 w444 w455 w492]
                tunnel: [w426 w430 w435 w438 w454 w491] -> w413
                tunnel: w412 -> [w423 w429 w434 w443 w457 w494]
                tunnel: [w425 w428 w433 w439 w456 w493] -> w415
                frame "False", Default {
                  n205 = VISA Write(VISA resource name=w424, write buffer="s4s", error in (no error)=w423) -> (VISA resource name out=w426:refnum<visa-resource-name>, error out=w425:errorcluster)  [unwired: 1 out]
                }
                frame "optomotorR" {
                  n206 = VISA Write(VISA resource name=w431, write buffer="s3r", error in (no error)=w429) -> (VISA resource name out=w430:refnum<visa-resource-name>, error out=w428:errorcluster)  [unwired: 1 out]
                }
                frame "optomotorL" {
                  n207 = VISA Write(VISA resource name=w436, write buffer="s3l", error in (no error)=w434) -> (VISA resource name out=w435:refnum<visa-resource-name>, error out=w433:errorcluster)  [unwired: 1 out]
                }
                frame "yt" {
                  n208 = local read "pattern"() -> (w442:u32)
                  n209 = VISA Write(VISA resource name=w444, write buffer="s1s", error in (no error)=w443) -> (VISA resource name out=w441:refnum<visa-resource-name>, error out=w440:errorcluster)  [unwired: 1 out]
                  n210 = case shown="9" w442 {
                    tunnel: w441 -> [w447 w451]
                    tunnel: w440 -> [w446 w450]
                    tunnel: [w446 w449] -> w439
                    tunnel: [w447 w448] -> w438
                    frame 0, Default {
                    }
                    frame 9 {
                      n211 = VISA Write(VISA resource name=w451, write buffer="D", error in (no error)=w450) -> (VISA resource name out=w448:refnum<visa-resource-name>, error out=w449:errorcluster)  [unwired: 1 out]
                    }
                  }
                }
                frame "sw" {
                  n212 = local read "pattern"() -> (w453:u32)
                  n213 = case shown="7" w453 {
                    tunnel: w457 -> [w458 w463 w479]
                    tunnel: [w458 w461 w478] -> w456
                    tunnel: w455 -> [w459 w464 w477]
                    tunnel: [w459 w462 w476] -> w454
                    frame 0, Default {
                    }
                    frame 8 {
                      n214 = local read "Sign"() -> (w460:bool)
                      n215 = case shown="False" w460 {
                        tunnel: w463 -> [w466 w473]
                        tunnel: [w465 w472] -> w461
                        tunnel: w464 -> [w468 w471]
                        tunnel: [w467 w470] -> w462
                        frame True {
                          n216 = VISA Write(VISA resource name=w468, write buffer="G", error in (no error)=w466) -> (VISA resource name out=w467:refnum<visa-resource-name>, error out=w465:errorcluster)  [unwired: 1 out]
                        }
                        frame False {
                          n217 = VISA Write(VISA resource name=w471, write buffer="B", error in (no error)=w473) -> (VISA resource name out=w470:refnum<visa-resource-name>, error out=w472:errorcluster)  [unwired: 1 out]
                        }
                      }
                    }
                    frame 7 {
                      n218 = local read "Sign"() -> (w475:bool)
                      n219 = case shown="True" w475 {
                        tunnel: w479 -> [w481 w488]
                        tunnel: [w480 w487] -> w478
                        tunnel: w477 -> [w483 w486]
                        tunnel: [w482 w485] -> w476
                        frame False {
                          n220 = VISA Write(VISA resource name=w483, write buffer="G", error in (no error)=w481) -> (VISA resource name out=w482:refnum<visa-resource-name>, error out=w480:errorcluster)  [unwired: 1 out]
                        }
                        frame True {
                          n221 = VISA Write(VISA resource name=w486, write buffer="B", error in (no error)=w488) -> (VISA resource name out=w485:refnum<visa-resource-name>, error out=w487:errorcluster)  [unwired: 1 out]
                        }
                      }
                    }
                  }
                }
                frame "fs" {
                  n222 = local read "pattern"() -> (w490:u32)
                  n223 = case shown="4" w490 {
                    tunnel: w494 -> [w495 w501 w506 w511 w516]
                    tunnel: [w495 w499 w504 w509 w514] -> w493
                    tunnel: w492 -> [w496 w500 w505 w510 w515]
                    tunnel: [w496 w498 w503 w508 w513] -> w491
                    frame 0, Default {
                    }
                    frame 3 {
                      n224 = VISA Write(VISA resource name=w500, write buffer="s3s", error in (no error)=w501) -> (VISA resource name out=w498:refnum<visa-resource-name>, error out=w499:errorcluster)  [unwired: 1 out]
                    }
                    frame 2 {
                      n225 = VISA Write(VISA resource name=w505, write buffer="s2s", error in (no error)=w506) -> (VISA resource name out=w503:refnum<visa-resource-name>, error out=w504:errorcluster)  [unwired: 1 out]
                    }
                    frame 1 {
                      n226 = VISA Write(VISA resource name=w510, write buffer="s1s", error in (no error)=w511) -> (VISA resource name out=w508:refnum<visa-resource-name>, error out=w509:errorcluster)  [unwired: 1 out]
                    }
                    frame 4 {
                      n227 = VISA Write(VISA resource name=w515, write buffer="s4s", error in (no error)=w516) -> (VISA resource name out=w513:refnum<visa-resource-name>, error out=w514:errorcluster)  [unwired: 1 out]
                    }
                  }
                }
              }
              n228 = feedback #1() -> (w414:errorcluster)  [unwired: 1 in]
              n229 = feedback-in #1(w415) -> ()
              "currentType" <- w407
            }
          }
          n230 = case shown="Error" w371 {
            selector: w371 -> [_ w403]
            frame No Error {
            }
            frame Error {
              n231 = Unbundle By Name(w403) -> ("source"=w402:string)
              n232 = property on="Stop Program" class="Bool (strict)"("Value"=TRUE) -> ()  [unwired: 2 in, 2 out]
              n233 = One Button Dialog(message=w402) -> ()  [unwired: 1 in, 1 out]
            }
          }
          n234 = local read "Stop Program"() -> (w368:bool)
          n235 = Send Notification(notification=w368, notifier=w372, error in (no error)=w371) -> (notifier out=w370:refnum<notifier>, error out=w369:errorcluster)
          n236 = Or(x=w369, y=w368) -> (x .or. y?=w367:bool)
        }
        n237 = Merge Errors(w73, w103, w146) -> (w72:errorcluster)
        n238 = Release Queue(queue=w84, error in (no error)=w72) -> (error out=w75:errorcluster)  [unwired: 1 in, 2 out]
        n239 = Release Notifier(notifier=w74, error in (no error)=w75) -> (error out=w71:errorcluster)  [unwired: 1 in, 2 out]
        n240 = VISA Write(VISA resource name=w94, write buffer="S", error in (no error)=w71) -> (VISA resource name out=w93:refnum<visa-resource-name>, error out=w95:errorcluster)  [unwired: 1 out]
        n241 = Close File(refnum=w102, error in=w95) -> (error out=w101:errorcluster)  [unwired: 1 out]
        n242 = call "rename_xml.vi"("error in"=w101, "xml"=w98, "csv"=w99) -> ("error out"=w100:errorcluster)  [unwired: 4 in]
        n243 = VISA Close(VISA resource name=w93, error in (no error)=w100) -> (error out=w126:errorcluster)
        n244 = call "labjack.vi"("error out"=w126, "Boolean"=FALSE, "Handle Out"=w121) -> ("error out 2"=w127:errorcluster, "Handle Out 2"=w125:i32)  [unwired: 6 in, 1 out]
        n245 = call "LJM_Close.vi"("error in"=w127, "Handle"=w125) -> ("error out"=w124:errorcluster)  [unwired: 9 in]
        "error out" <- w124
        n246 = call "LJM_ErrorToString.vi"("error in"=w124) -> ("String"=→"Error String":string)  [unwired: 10 in]
      }
    }
    n247 = local write "millisecond timer value 2"("millisecond timer value 2") -> ()
    n248 = Wait (ms)(milliseconds to wait=u32 5) -> ()  [unwired: 1 out]
    n249 = local read "Stop Program"() -> (w67:bool)
  }
  n250 = local read "deleted portion"() -> (→"deleted portion":u8[])
  n251 = local read "Output"() -> (→"Output":bool)
  n252 = local read "Sign"() -> (→"Sign":bool)
  n253 = local read "PWM"() -> (→"PWM":bool)
  n254 = local read "data"() -> (→"data":bool)
  n255 = local read "Read"() -> (→"Read":bool)
  n256 = flat-sequence {
    tunnel: w10 -> [w576]
    tunnel: [w576] -> w9
    tunnel: w9 -> [w577]
    frame #0 {
      n257 = Not(x=w576) -> (.not. x?=w575:bool)
      n258 = local write "Stop Program"(w575) -> ()
    }
    frame #1 {
      n259 = Stop(stop? (T)=w577) -> ()
    }
  }
  "Progress" <- 0.0 ("Slide")
  "Time" <- 0.0 ("Progress 2")
